vi "SHUTTER_TYPE - Type.vi"(8 "error in (no error)":errorcluster) -> (0 "error out":errorcluster, 3 "SHUTTER_TYPE_VALUE":i32)   [LabVIEW 2013]
doc: "<b>Buffer policy settings can be only unsafe in xiAPI LabVIEW library</b>\nUNSAFE : User gets pointer to internally allocated circle buffer and data may be overwritten by device.\nSAFE : Data from device will be copied to user allocated buffer or xiApi allocated memory."
uses:
  SHUTTER_TYPE.ctl
  C:/Projects/Cameras3.x/xiLib/xiLIB_64bit/xiLIB/xiCamLib/API/x64/xiApi.NETX64.dll
  xiLIB_64bit/xiLIB/xiCamLib/API/x64/xiApi.NETX64.dll
panel:
  in  "SHUTTER_TYPE":T1
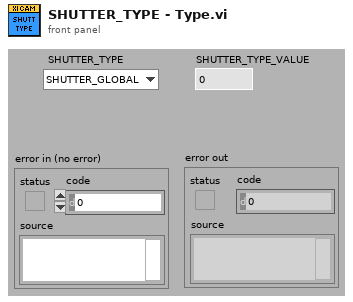
[diagram p1: front panel]
types:
  T1 = typedef "SHUTTER_TYPE.ctl" = enum16{"SHUTTER_GLOBAL", "SHUTTER_ROLLING", "SHUTTER_GLOBAL_RESET_RELEASE"}
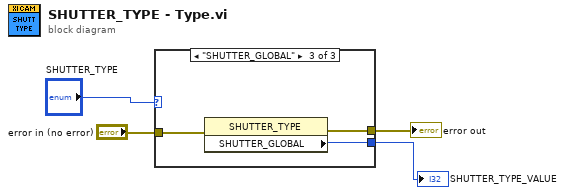
[diagram p0: block diagram]
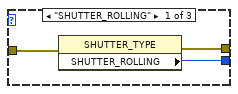
[diagram p2: hidden frame]
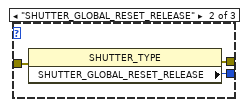
[diagram p3: hidden frame]
diagram:
  n1 = case shown="\"SHUTTER_GLOBAL\"" "SHUTTER_TYPE" {
    tunnel: "error in (no error)" -> [w7 w10 w13]
    tunnel: [w6 w9 w12] -> w3
    tunnel: [w5 w8 w11] -> w2
    frame "SHUTTER_ROLLING" {
      n2 = property class="SHUTTER_TYPE"(error in=w7) -> (error out=w6:errorcluster, "SHUTTER_ROLLING"=w5:i32)  [unwired: 1 in, 1 out]
    }
    frame "SHUTTER_GLOBAL_RESET_RELEASE" {
      n3 = property class="SHUTTER_TYPE"(error in=w10) -> (error out=w9:errorcluster, "SHUTTER_GLOBAL_RESET_RELEASE"=w8:i32)  [unwired: 1 in, 1 out]
    }
    frame "SHUTTER_GLOBAL" {
      n4 = property class="SHUTTER_TYPE"(error in=w13) -> (error out=w12:errorcluster, "SHUTTER_GLOBAL"=w11:i32)  [unwired: 1 in, 1 out]
    }
  }
  "error out" <- w3
  "SHUTTER_TYPE_VALUE" <- w2
